vi "Is Clear.vi"(10 "Direction":T1, 11 "Maze":i32[](array[numeric])) -> (1 "Can Move?":bool, 2 "Direction Out":T1, 3 "Maze":i32[](array[numeric]))   [LabVIEW 2015, in "Rain.lvclass"]
uses:
  Rain.lvclass
  Type Defs/Direction Enum.ctl
  Type Defs/SB Type Defs.lvlib
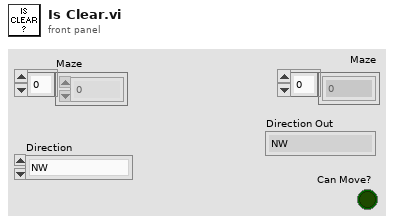
[diagram p1: front panel]
types:
  T1 = typedef "SB Type Defs.lvlib/Direction Enum.ctl" = enum16{"NW", "N", "NE", "E", "SE", "S", "SW", "W"}
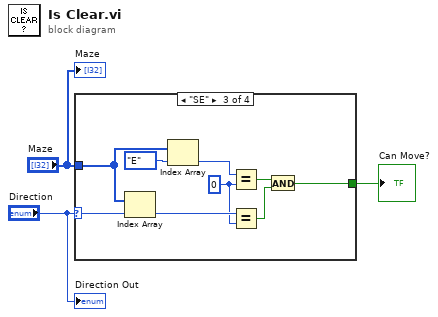
[diagram p0: block diagram]
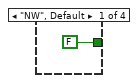
[diagram p2: hidden frame]
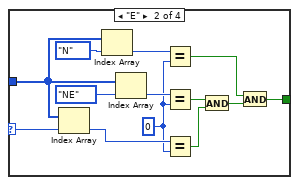
[diagram p3: hidden frame]
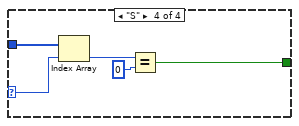
[diagram p4: hidden frame]
diagram:
  n1 = case shown="\"SE\"" "Direction" {
    selector: "Direction" -> [_ w16 w25 w29]
    tunnel: "Maze" -> [_ w12 w22 w28]
    tunnel: [FALSE w5 w18 w27] -> w2
    frame "NW", Default {
    }
    frame "E" {
      w10 = 0
      n2 = Index Array(array=w12, index=w16) -> (element=w17:i32)
      n3 = Index Array(array=w12, index=Direction_Enum."N" ("Direction 2")) -> (element=w11:i32)
      n4 = Index Array(array=w12, index=Direction_Enum."NE" ("Direction 2")) -> (element=w15:i32)
      n5 = Equal?(x=w11, y=w10) -> (x = y?=w6:bool)
      n6 = Equal?(x=w15, y=w10) -> (x = y?=w8:bool)
      n7 = Equal?(x=w17, y=w10) -> (x = y?=w9:bool)
      n8 = And(x=w8, y=w9) -> (x .and. y?=w7:bool)
      n9 = And(x=w6, y=w7) -> (x .and. y?=w5:bool)
    }
    frame "SE" {
      w21 = 0
      n10 = Index Array(array=w22, index=w25) -> (element=w26:i32)
      n11 = Index Array(array=w22, index=Direction_Enum."E" ("Direction 2")) -> (element=w23:i32)
      n12 = Equal?(x=w23, y=w21) -> (x = y?=w19:bool)
      n13 = Equal?(x=w26, y=w21) -> (x = y?=w20:bool)
      n14 = And(x=w19, y=w20) -> (x .and. y?=w18:bool)
    }
    frame "S" {
      n15 = Index Array(array=w28, index=w29) -> (element=w31:i32)
      n16 = Equal?(x=w31, y=0) -> (x = y?=w27:bool)
    }
  }
  "Can Move?" <- w2
  "Maze" <- "Maze"
  "Direction Out" <- "Direction"
